vi "Triggered Acquisition Demo.vi"() -> ()   [LabVIEW 2015]
uses:
  <vilib>/DAQmx/write.llb/DAQmx Write (Analog 1D DBL 1Chan NSamp).vi
  <vilib>/DAQmx/read.llb/DAQmx Read (Analog 1D DBL 1Chan NSamp).vi
  <vilib>/DAQmx/miscellaneous.llb/DAQmx Fill In Error Info.vi
panel:
  out "Trial number":i32
  out "Start time (ms)":u32
  out "finished":bool
  out "Graph":dbl[](graph)
  in  "Gate":T1={"Active"=TRUE, "Delay (ms)"=20.0, "Width (ms)"=100.0, "Ramp (ms)"=5.0}
  out "Abort":bool
  in  "START":bool
  in  "RETURN":bool
  in  "STOP":bool
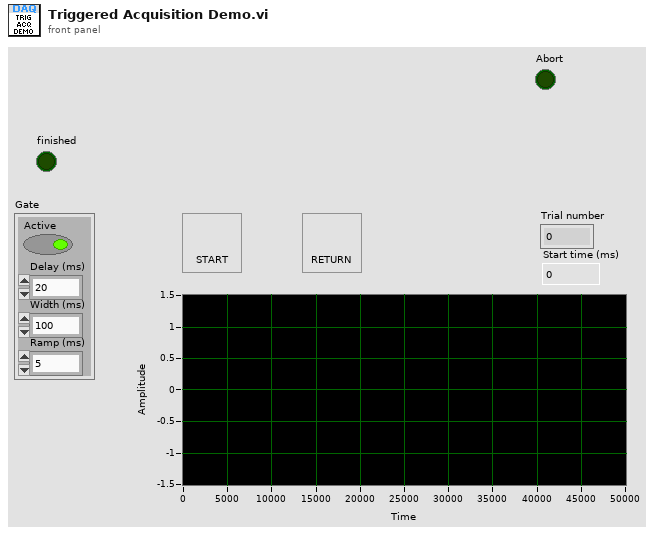
[diagram p1: front panel]
types:
  T1 = cluster{"Active":bool, "Delay (ms)":dbl, "Width (ms)":dbl, "Ramp (ms)":dbl}
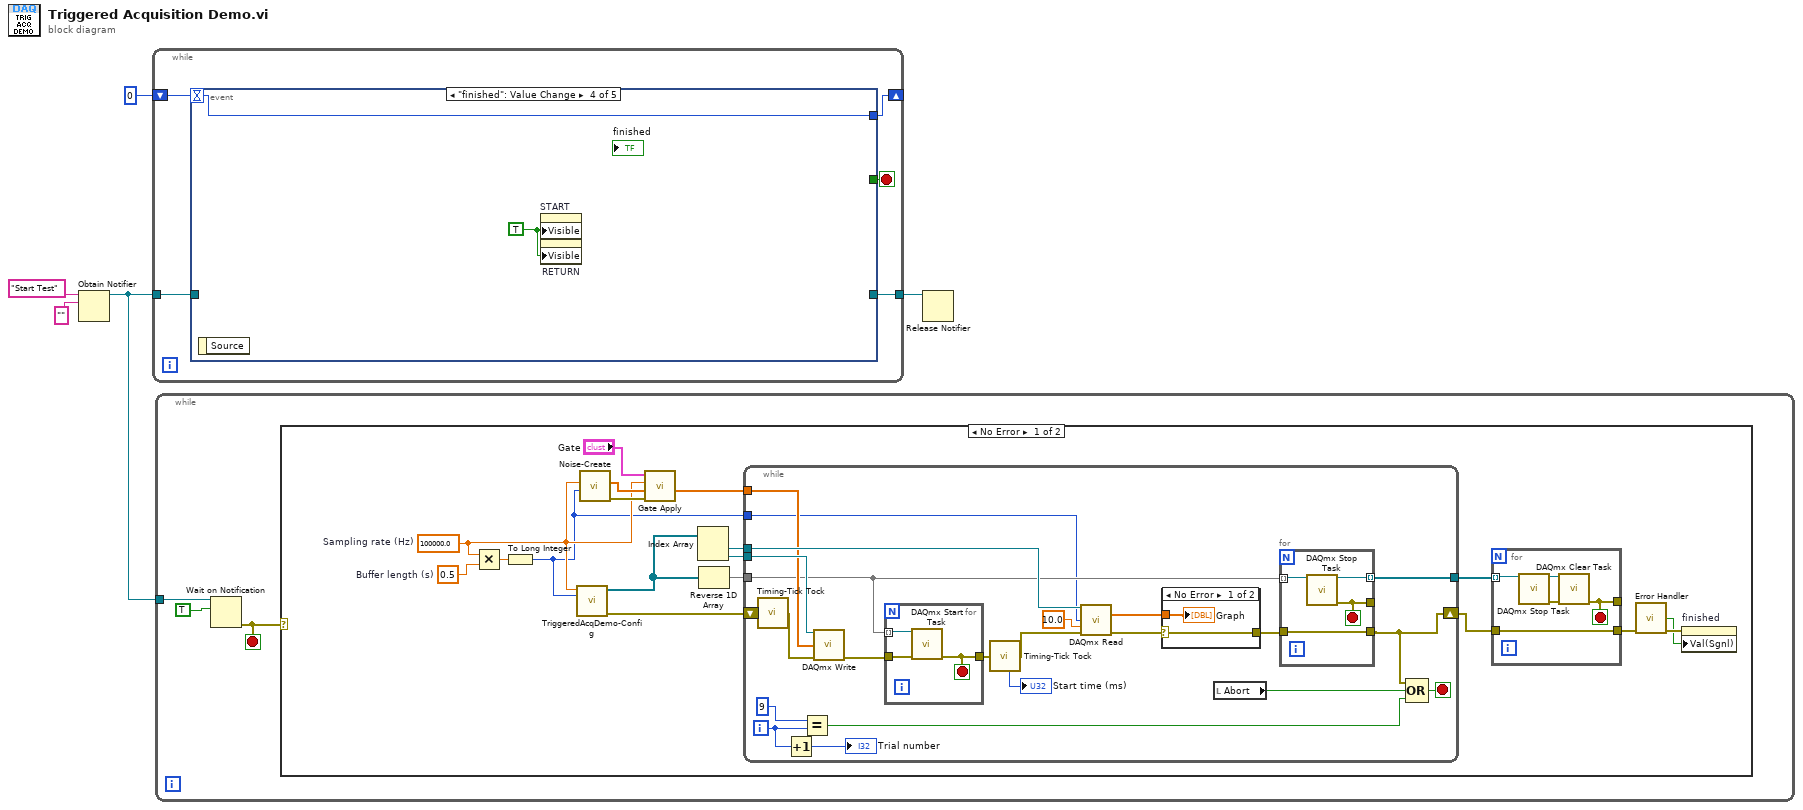
[diagram p0: block diagram]
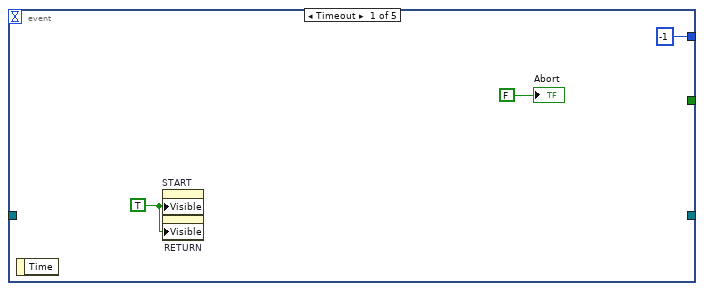
[diagram p4: hidden frame]
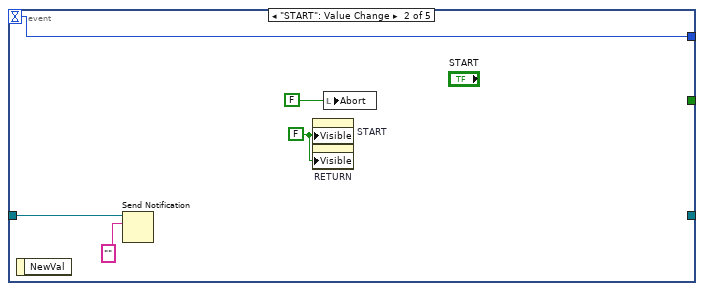
[diagram p5: hidden frame]
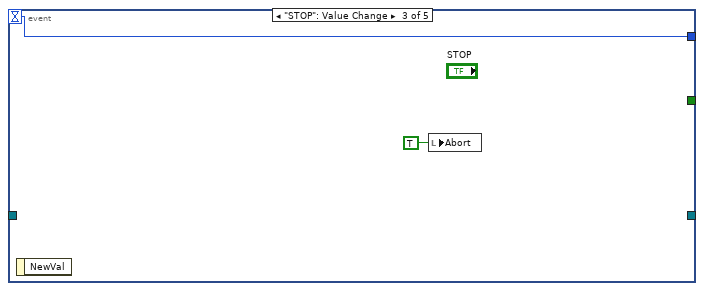
[diagram p6: hidden frame]
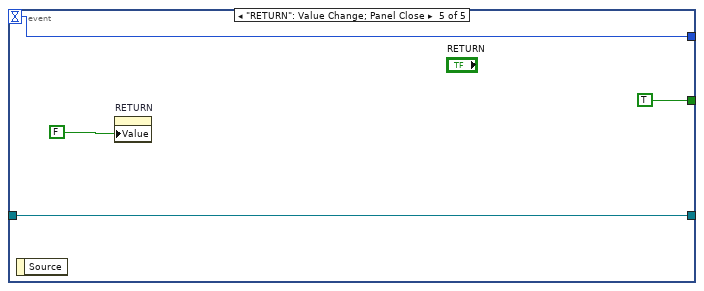
[diagram p7: hidden frame]
diagram:
  n1 = Obtain Notifier(name (unnamed)="Start Test", notification data type="") -> (notifier out=w5:refnum<notifier>)  [unwired: 2 in, 2 out]
  n2 = while {
    tunnel: w5 -> [w10]
    tunnel: [w8] -> w4
    shift-right: [w6] -> _
    shift-left: 0 -> [w7]
    stop <- w9 stop-if-true
    n3 = event shown="[3] \"finished\": Value Change" {
      selector: _ -> [_ _ _ _ _]
      dyn-events: _ -> [_ _ _ _ _]
      timeout: w7 -> [_ w16 w19 w22 w24]
      tunnel: w10 -> [_ w17 _ _ w25]
      tunnel: [_ _ _ _ TRUE] -> w9
      tunnel: [_ _ _ _ w25] -> w8
      tunnel: [-1 w16 w19 w22 w24] -> w6
      event Timeout {
        w11 = TRUE ("Visible")
        n4 = event-data() -> ()  [unwired: 1 in, 1 out]
        n5 = property on="START" class="Bool"("Visible"=w11) -> ()  [unwired: 2 in, 2 out]
        n6 = property on="RETURN" class="Bool (strict)"("Visible"=w11) -> ()  [unwired: 2 in, 2 out]
        "Abort" <- FALSE ("Abort")
      }
      event "START": Value Change {
        w14 = FALSE ("Visible")
        n7 = event-data() -> ()  [unwired: 1 in, 1 out]
        n8 = Send Notification(notification="", notifier=w17) -> ()  [unwired: 1 in, 2 out]
        n9 = property on="START" class="Bool"("Visible"=w14) -> ()  [unwired: 2 in, 2 out]
        n10 = property on="RETURN" class="Bool (strict)"("Visible"=w14) -> ()  [unwired: 2 in, 2 out]
        n11 = local write "Abort"(FALSE ("Global Abort")) -> ()
      }
      event "STOP": Value Change {
        n12 = event-data() -> ()  [unwired: 1 in, 1 out]
        n13 = local write "Abort"(TRUE ("Global Abort")) -> ()
      }
      event "finished": Value Change {
        w21 = TRUE ("Visible")
        n14 = event-data() -> ()  [unwired: 1 in, 1 out]
        n15 = property on="START" class="Bool"("Visible"=w21) -> ()  [unwired: 2 in, 2 out]
        n16 = property on="RETURN" class="Bool (strict)"("Visible"=w21) -> ()  [unwired: 2 in, 2 out]
      }
      event "RETURN": Value Change; Panel Close {
        n17 = event-data() -> ()  [unwired: 1 in, 1 out]
        n18 = property on="RETURN" class="Bool (strict)"("Value"=FALSE) -> ()  [unwired: 2 in, 2 out]
      }
    }
  }
  n19 = while {
    tunnel: w5 -> [w28]
    stop <- w27 stop-if-true
    n20 = Wait on Notification(notifier=w28, ignore previous (F)=TRUE) -> (error out=w27:errorcluster)  [unwired: 2 in, 3 out]
    n21 = case shown="No Error" w27 {
      frame No Error {
        w44 = 0.5  # Buffer length (s)
        w42 = 100000.0  # Sampling rate (Hz)
        n22 = Multiply(x=w42, y=w44) -> (x*y=w43:dbl)
        n23 = To Long Integer(number=w43) -> (32bit integer=w35:i32)
        n24 = call "TriggeredAcqDemo-Config.vi"("Npts"=w35, "Fs"=w42) -> ("error out"=w38:errorcluster, "tasks"=w39:refnum<k21>[])  [unwired: 8 in]
        n25 = call "Noise-Create.vi"("Npts"=w35, "Sampling Rate (Hz)"=w42) -> ("error out"=w45:errorcluster, "Waveform"=w46:dbl[])  [unwired: 7 in, 1 out]
        n26 = call "Gate Apply.vi"("error in (no error)"=w45, "Waveform in"=w46, "Sampling Rate (Hz)"=w42, "Gate Control"="Gate") -> ("Gated waveform"=w36:dbl[])  [unwired: 6 in, 1 out]
        n27 = Index Array(array=w39) -> (element #1=w41:refnum<k21>, element #2=w37:refnum<k21>)  [unwired: 2 in]
        n28 = Reverse 1D Array(array=w39) -> (reversed array=w32:refnum<k21>[])
        n29 = while {
          tunnel: w32 -> [w58]
          tunnel: [w55] -> w40
          tunnel: w41 -> [w65]
          shift-right: [w56] -> w33
          shift-left: w38 -> [w53]
          tunnel: w37 -> [w63]
          tunnel: w36 -> [w62]
          tunnel: w35 -> [w54]
          i -> [w68]
          stop <- w70 stop-if-true
          n30 = call "Timing-Tick Tock.vi"("error in (no error)"=w53) -> ("error out"=w52:errorcluster)  [unwired: 5 in, 1 out]
          n31 = Increment(x=w68) -> (x+1=→"Trial number":i32)
          n32 = Equal?(x=9, y=w68) -> (x = y?=w66:bool)
          n33 = call-poly <vilib>:"DAQmx Write.vi"("task/channels in"=w63, "data"=w62, "error in"=w52) -> ("error out"=w64:errorcluster)  [unwired: 10 in, 2 out]
          n34 = for {
            tunnel: w64 -> [w80]
            tunnel: w58 -> [w79] mode=indexing
            tunnel: [w78] -> w51
            stop <- w78 stop-if-true
            n35 = call <vilib>:"DAQmx Start Task.vi"("task/channels in"=w79, "error in"=w80) -> ("error out"=w78:errorcluster)  [unwired: 12 in, 1 out]
          }
          n36 = call "Timing-Tick Tock.vi"("error in (no error)"=w51) -> ("Elapsed time (ms)"=→"Start time (ms)":u32, "error out"=w50:errorcluster)  [unwired: 5 in]
          n37 = call-poly <vilib>:"DAQmx Read.vi"("task/channels in"=w65, "number of samples per channel"=w54, "timeout"=10.0, "error in"=w50) -> ("data"=w59:dbl[], "error out"=w60:errorcluster)  [unwired: 9 in, 1 out]
          n38 = case shown="No Error" w60 {
            selector: w60 -> [w76 w77]
            tunnel: [w76 w77] -> w57
            tunnel: w59 -> [w75 _]
            frame No Error {
              "Graph" <- w75
            }
            frame Error {
            }
          }
          n39 = local read "Abort"() -> (w69:bool)
          n40 = for {
            tunnel: w58 -> [w74] mode=indexing
            tunnel: [w72] -> _
            tunnel: [w73] -> w56
            tunnel: w57 -> [w73]
            tunnel: [w71] -> w55 mode=indexing
            stop <- w72 stop-if-true
            n41 = call <vilib>:"DAQmx Stop Task.vi"("task/channels in"=w74) -> ("task out"=w71:refnum<k21>, "error out"=w72:errorcluster)  [unwired: 13 in]
          }
          n42 = Compound Arithmetic op=OR(w56, w69, w66) -> (w70:bool)
        }
        n43 = for {
          tunnel: w40 -> [w85] mode=indexing
          tunnel: [w82] -> _
          tunnel: [w81] -> w34
          tunnel: w33 -> [w81]
          stop <- w82 stop-if-true
          n44 = call <vilib>:"DAQmx Stop Task.vi"("task/channels in"=w85) -> ("task out"=w84:refnum<k21>, "error out"=w83:errorcluster)  [unwired: 13 in]
          n45 = call <vilib>:"DAQmx Clear Task.vi"("task in"=w84, "error in"=w83) -> ("error out"=w82:errorcluster)  [unwired: 13 in]
        }
        n46 = call "Error Handler.vi"("error in (no error)"=w34) -> ("error?"=w30:bool, "No Error"=w31:errorcluster)  [unwired: 13 in]
        n47 = property on="finished" class="Bool (strict)"(error in=w31, "Val(Sgnl)"=w30) -> ()  [unwired: 1 in, 2 out]
      }
      frame Error {
      }
    }
  }
  n48 = Release Notifier(notifier=w4) -> ()  [unwired: 2 in, 3 out]
